vi "Initialize.vi"(5 "ID or SN":string, 7 "Test File Path":path, 9 "INI File Path":path, 11 "error in (no error)":errorcluster) -> (4 "BFECC out":refnum<class "BFECC.lvclass">, 15 "error out":errorcluster)   [LabVIEW 2018, in "BFECC.lvlib" / "BFECC.lvclass"]
uses:
  BFECC.lvclass
  BFECC.lvclass/BFECC.ctl
  AME Test Engineering/LabVIEW/PPLs/Configuration/Configuration.lvlibp/Configuration.lvclass
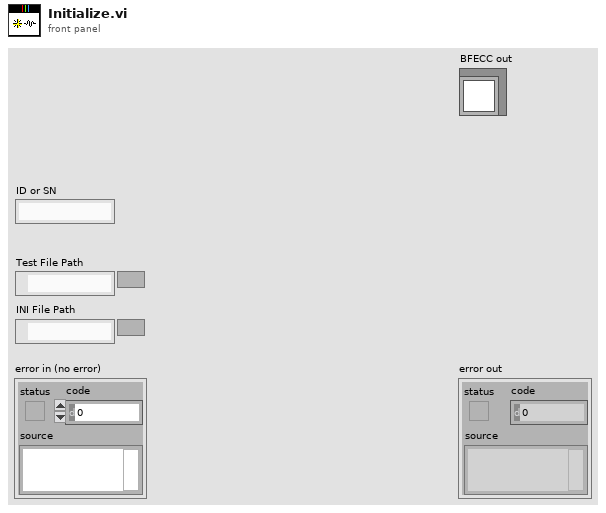
[diagram p1: front panel]
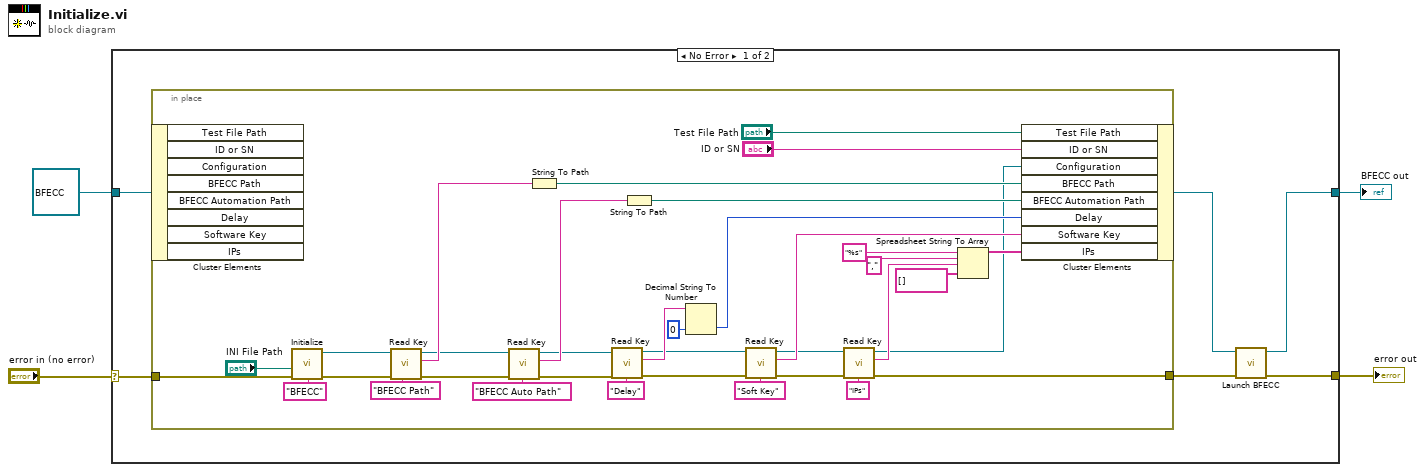
[diagram p0: block diagram]
diagram:
  n1 = case shown="No Error" "error in (no error)" {
    selector: "error in (no error)" -> [w9 w47]
    tunnel: [w6 w47] -> w3
    tunnel: [w5 w46] -> w1
    tunnel: refnum<class "BFECC.lvclass"> refnum ("BFECC in") -> [w10 w46]
    frame No Error {
      n2 = in-place {
        in-place-border: w9 -> [w45]
        in-place-border: [w17] -> w7
        n3 = in-place-cluster #1(w10) -> ()  [unwired: 8 out]
        n4 = call "Initialize.vi"("error in"=w45, "INI File Path"="INI File Path", "Device"="BFECC") -> ("error out"=w42:errorcluster, "Configuration out"=w41:refnum<class "Configuration.lvclass">)  [unwired: 7 in]
        n5 = call "Read Key.vi"("Key:"="BFECC Path", "error in"=w42, "Configuration in"=w41) -> ("error out"=w36:errorcluster, "Value"=w39:string, "Configuration out"=w35:refnum<class "Configuration.lvclass">)  [unwired: 6 in]
        n6 = call "Read Key.vi"("Key:"="BFECC Auto Path", "error in"=w36, "Configuration in"=w35) -> ("error out"=w31:errorcluster, "Value"=w34:string, "Configuration out"=w30:refnum<class "Configuration.lvclass">)  [unwired: 6 in]
        n7 = String To Path(string=w39) -> (path=w38:path)
        n8 = call "Read Key.vi"("Key:"="Delay", "error in"=w31, "Configuration in"=w30) -> ("error out"=w25:errorcluster, "Value"=w29:string, "Configuration out"=w24:refnum<class "Configuration.lvclass">)  [unwired: 6 in]
        n9 = String To Path(string=w34) -> (path=w33:path)
        n10 = Decimal String To Number(string=w29, default (0L)=u32 0 ("default (0 I32)")) -> (number=w27:u32)  [unwired: 1 in, 1 out]
        n11 = call "Read Key.vi"("Key:"="Soft Key", "error in"=w25, "Configuration in"=w24) -> ("error out"=w21:errorcluster, "Value"=w23:string, "Configuration out"=w20:refnum<class "Configuration.lvclass">)  [unwired: 6 in]
        n12 = call "Read Key.vi"("Key:"="IPs", "error in"=w21, "Configuration in"=w20) -> ("error out"=w17:errorcluster, "Value"=w15:string, "Configuration out"=w12:refnum<class "Configuration.lvclass">)  [unwired: 6 in]
        n13 = Spreadsheet String To Array(delimiter (Tab)=",", format string="%s", spreadsheet string=w15, array type (2D Dbl)=string[] []) -> (array=w18:string[])
        n14 = in-place-cluster #1("Test File Path"="Test File Path", "ID or SN"="ID or SN", "Configuration"=w12, "BFECC Path"=w38, "BFECC Automation Path"=w33, "Delay"=w27, "Software Key"=w23, "IPs"=w18) -> (w8:refnum<class "BFECC.lvclass">)
      }
      n15 = call "Launch BFECC.vi"("error in (no error)"=w7, "BFECC in"=w8) -> ("error out"=w6:errorcluster, "BFECC out"=w5:refnum<class "BFECC.lvclass">)  [unwired: 8 in]
    }
    frame Error {
    }
  }
  "error out" <- w3
  "BFECC out" <- w1
